vi "test_abs_activity.vi"() -> ()   [LabVIEW 2017]
doc: "Minimal example that demonstrates functions implemented in the SorpPropLib for absorption working pairs based on the acitvity approach."
panel:
  in  "Molar volume of second component in m3/mol (Input)":dbl=-1.0
  in  "Molar volume of first component in m3/mol (Input)":dbl=-1.0
  out "Activity coefficient of first component":cluster{dbl[], dbl[]}[](graph)=[{[1000.0, 1001.0, 1002.0, 1003.0, 1004.0, 1005.0, 1006.0, 1007.0, 1008.0, 1009.0], [6.057709632538217, 6.057704701039578, 6.057699769539269, 6.057694838037295, 6.05768990653365, 6.05768497502834, 6.057680043521361, 6.0576751120127135, 6.0576701805024005, 6.057665248990417]}]
  out "Pressure":cluster{dbl[], dbl[]}[](graph)=[{[1000.0, 1001.0, 1002.0, 1003.0, 1004.0, 1005.0, 1006.0, 1007.0, 1008.0, 1009.0], [999.9999999999999, 1001.0, 1002.0, 1003.0000000000001, 1004.0, 1005.0, 1006.0, 1007.0, 1008.0, 1009.0]}]
  out "Mole fraction in liquid phase":cluster{dbl[], dbl[]}[](graph)=[{[1000.0, 1001.0, 1002.0, 1003.0, 1004.0, 1005.0, 1006.0, 1007.0, 1008.0, 1009.0], [0.00023489755625797214, 0.00023513264523250375, 0.00023536773458986628, 0.0002356028243300607, 0.00023583791445308842, 0.00023607300495895024, 0.0002363080958476475, 0.0002365431871191813, 0.00023677827877355265, 0.0002370133708107629]}]
  in  "WorkingPair (Input)":T1={"no_iso"=1, "no_p_sat"=1, "path_db"="D:\\Driesel\\SorpLibLocal\\labview_wrapper\\data\\json\\sorpproplib.json", "wp_as"="lubricant", "wp_st"="POE", "wp_iso"="WilsonFixedDl", "wp_rf"="R-134a", "rf_rhol"="SaturatedLiquidDensity_EoS1", "no_rhol"=1, "rf_psat"="VaporPressure_EoS1"}
  in  "Temperature in K (Input)":dbl=300.0
  in  "Pressure in Pa (Input)":dbl=500000.0
  # "Increase pressure by 10 Pa in steps of 1 Pa."
  # "Selecting -1: Constant molar volumes stored in data base are used for calculations!"
  # "Path to database"
  # "Name of sorbent"
  # "Name of sub-type of sorbent"
  # "Name of refrigerant"
  # "Name of isotherm"
  # "ID of isotherm"
  # "Name of calculation approach for vapor pressure"
  # "ID of vapor pressure equation"
  # "Name of calculation approach for liquid density"
  # "ID of liquid density equation"
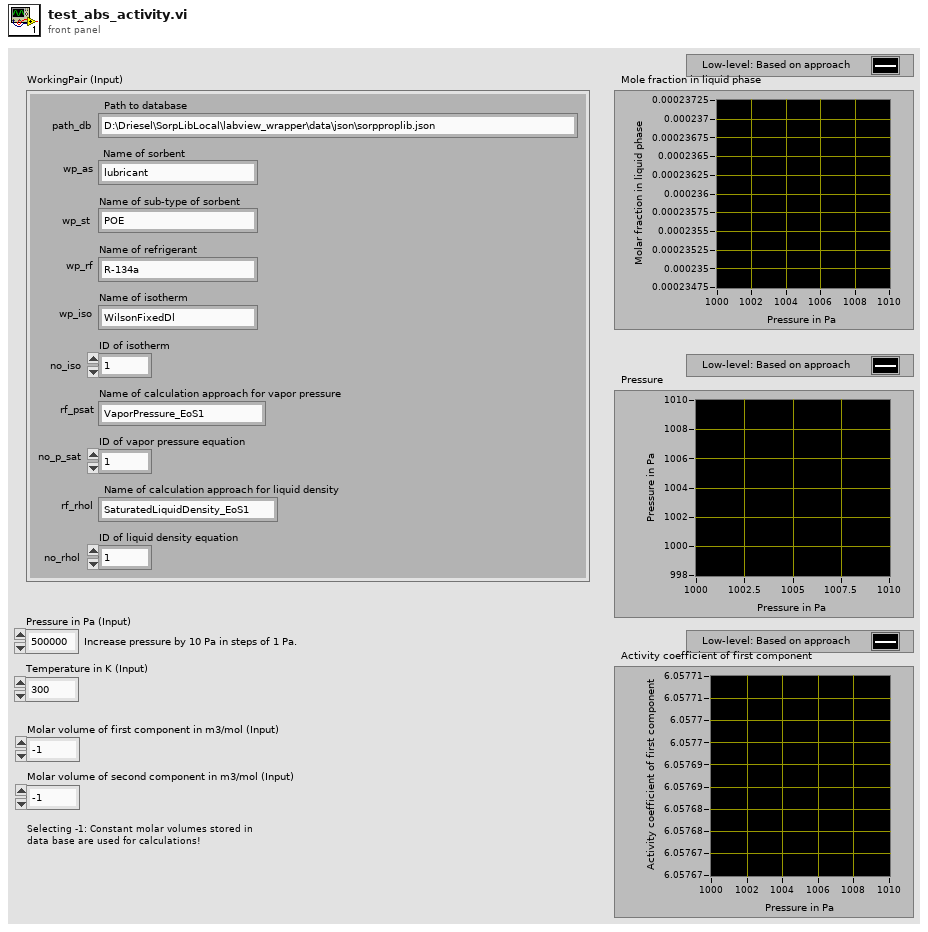
[diagram p1: front panel]
types:
  T1 = cluster{"no_iso":i32, "no_p_sat":i32, "path_db":string, "wp_as":string, "wp_st":string, "wp_iso":string, "wp_rf":string, "rf_rhol":string, "no_rhol":i32, "rf_psat":string}
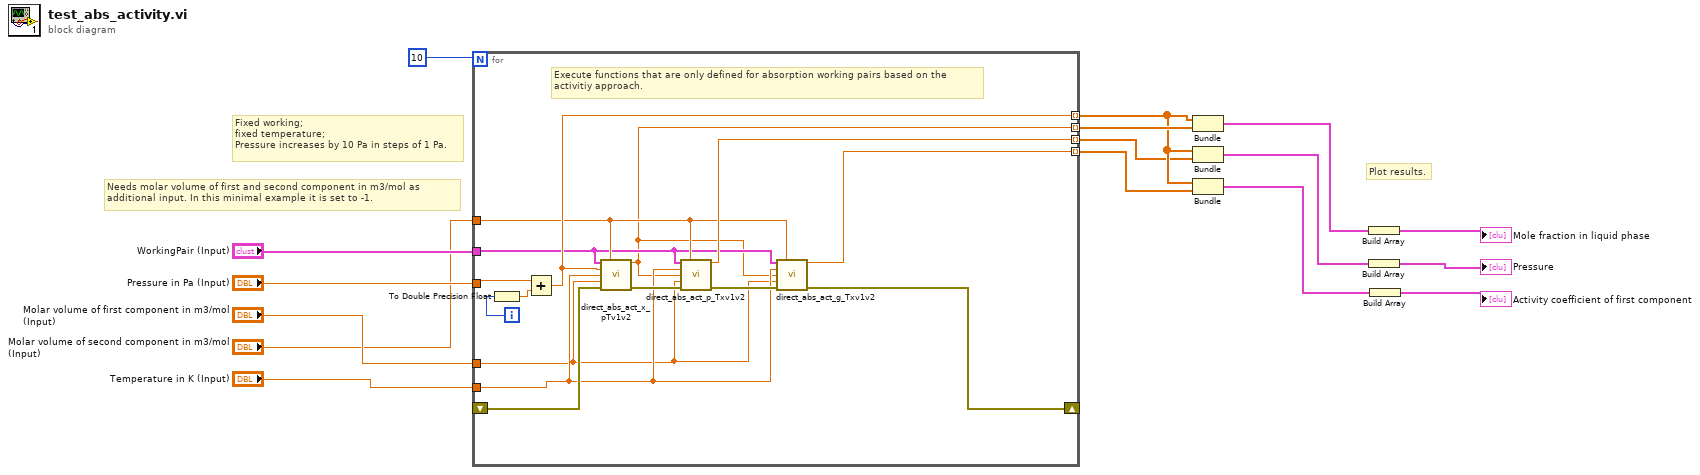
[diagram p0: block diagram]
diagram:
  # "Needs molar volume of first and second component in m3/mol as \nadditional input. In this minimal example it is set to -1."
  # "Plot results."
  # "Fixed working;\nfixed temperature;\nPressure increases by 10 Pa in steps of 1 Pa."
  n1 = for {
    N: 10 -> [_]
    tunnel: "Pressure in Pa (Input)" -> [w31]
    tunnel: "Temperature in K (Input)" -> [w20]
    tunnel: "WorkingPair (Input)" -> [w21]
    shift-right: [w23] -> _
    shift-left: _ -> [w28]
    tunnel: [w17] -> w11 mode=indexing
    tunnel: [w27] -> w13 mode=indexing
    tunnel: [w18] -> w14 mode=indexing
    tunnel: [w26] -> w12 mode=indexing
    tunnel: "Molar volume of first component in m3/mol (Input)" -> [w19]
    tunnel: "Molar volume of second component in m3/mol (Input)" -> [w22]
    i -> [w30]
    # "Execute functions that are only defined for absorption working pairs based on the\nactivitiy approach."
    n2 = To Double Precision Float(number=w30) -> (double precision float=w29:dbl)
    n3 = Add(x=w31, y=w29) -> (x+y=w27:dbl)
    n4 = call "direct_abs_act_x_pTv1v2.vi"("WorkingPair (Input)"=w21, "Molar volume of second component in m3/mol (Input)"=w22, "Pressure p_Pa in Pa (Input)"=w27, "Temperature in K (Input)"=w20, "Molar volume of first component in m3/mol (Input)"=w19, "Error (Input)"=w28) -> ("Mole fraction in liquid phase in mol/mol (Output)"=w18:dbl, "Error (Output)"=w25:errorcluster)  [unwired: 8 in]
    n5 = call "direct_abs_act_p_Txv1v2.vi"("WorkingPair (Input)"=w21, "Molar volume of second component in m3/mol (Input)"=w22, "Temperature in K (Input)"=w20, "Mole fraction in liquid phase in mol/mol (Input)"=w18, "Molar volume of first component in m3/mol (Input)"=w19, "Error (Input)"=w25) -> ("Pressure in Pa (Output)"=w26:dbl, "Error (Output)"=w24:errorcluster)  [unwired: 8 in]
    n6 = call "direct_abs_act_g_Txv1v2.vi"("WorkingPair (Input)"=w21, "Molar volume of second component in m3/mol (Input)"=w22, "Temperature in K (Input)"=w20, "Mole fraction in liquid phase in mol/mol (Input)"=w18, "Molar volume of first component in m3/mol (Input)"=w19, "Error (Input)"=w24) -> ("Activity coefficient of first component (Output)"=w17:dbl, "Error (Output)"=w23:errorcluster)  [unwired: 8 in]
  }
  n7 = Bundle(w13, w14) -> (w10:cluster{dbl[], dbl[]})  [unwired: 1 in]
  n8 = Bundle(w13, w12) -> (w9:cluster{dbl[], dbl[]})  [unwired: 1 in]
  n9 = Bundle(w13, w11) -> (w8:cluster{dbl[], dbl[]})  [unwired: 1 in]
  n10 = Build Array(w10) -> (→"Mole fraction in liquid phase":cluster{dbl[], dbl[]}[])
  n11 = Build Array(w9) -> (→"Pressure":cluster{dbl[], dbl[]}[])
  n12 = Build Array(w8) -> (→"Activity coefficient of first component":cluster{dbl[], dbl[]}[])
